vi "TDC_analyseHbtFunction.vi"(8 "Error In":errorcluster, 10 "Buffer Size":i32, 11 "Function":u64) -> (0 "Error Out":errorcluster, 1 "Values":dbl[](array[numeric]), 2 "Index Offset":i32, 3 "Bin Width":i32, 5 "Size":i32, 7 "Capacity":i32)   [LabVIEW 2011]
uses:
  tdcbase.dll
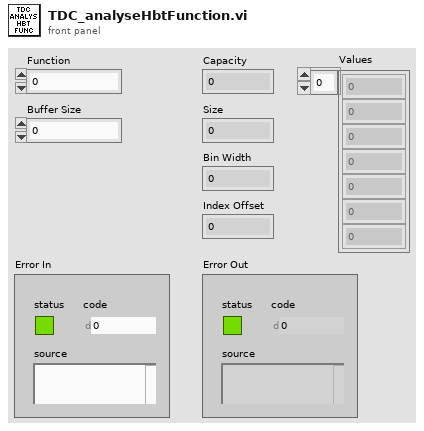
[diagram p1: front panel]
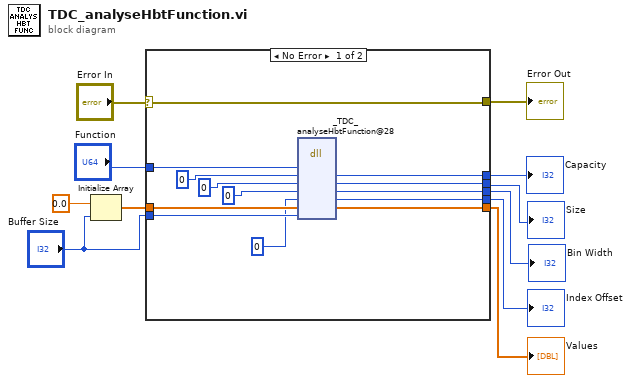
[diagram p0: block diagram]
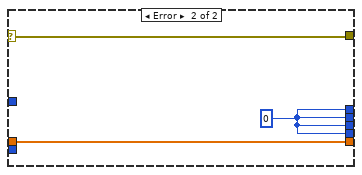
[diagram p2: hidden frame]
diagram:
  n1 = Initialize Array(0.0, "Buffer Size") -> (w7:dbl[])
  n2 = case shown="No Error" "Error In" {
    selector: "Error In" -> [w12 w27]
    tunnel: [w12 w27] -> w10
    tunnel: "Function" -> [w24 _]
    tunnel: w7 -> [w23 w25]
    tunnel: [w22 w25] -> w2
    tunnel: [w21 w26] -> w6
    tunnel: "Buffer Size" -> [w20 _]
    tunnel: [w19 w26] -> w5
    tunnel: [w18 w26] -> w4
    tunnel: [w17 w26] -> w3
    frame No Error {
      n3 = dll-call lib="X:/tdcbase.dll" fn="_TDC_analyseHbtFunction@28"("fct"=w24, "capacity"=0, "size"=0, "binWidth"=0, "iOffset"=0, "values"=w23, "bufSize"=w20) -> ("capacity"=w21:i32, "size"=w19:i32, "binWidth"=w18:i32, "iOffset"=w17:i32, "values"=w22:dbl[])  [unwired: 6 in, 2 out]
    }
    frame Error {
      w26 = 0
    }
  }
  "Error Out" <- w10
  "Capacity" <- w6
  "Index Offset" <- w3
  "Bin Width" <- w4
  "Size" <- w5
  "Values" <- w2
